vi "reward_behavior_michelle_visjitter_conswinAdapt_enticefx_TSLog_VF_forrecording.vi"() -> ()   [LabVIEW 2019]
doc: "The myRIO Project template acquires acceleration data from the onboard accelerometer and displays the changes of acceleration values in a waveform chart."
uses:
  <vilib>/Analysis/Matrix/Datatypes/RealMatrix.ctl
  <vilib>/myRIO/Instrument Drivers/Onboard IO/DIO/typedefs/DIO Reference.ctl
  <vilib>/myRIO/Common/Instrument Driver Framework/Utilities/typedefs/myRIO Generic Hardware Reference.ctl
  <vilib>/myRIO/Common/Instrument Driver Framework/Utilities/typedefs/Hardware Version Enum.ctl
  <vilib>/myRIO/Common/Instrument Driver Framework/Utilities/typedefs/myRIO v1.0 Reference.ctl
  <vilib>/myRIO/Common/Instrument Driver Framework/Utilities/typedefs/Generic FPGA Reference.ctl
  <vilib>/myRIO/Common/Instrument Driver Framework/myRIO v1.0/DIO/typedefs/DIO Channels List.ctl
  <vilib>/myRIO/Common/Instrument Driver Framework/myRIO v1.0/DIO/typedefs/DIO Channels Enum.ctl
  <vilib>/userdefined/High Color/nirio_resource_hc.ctl
  <vilib>/myRIO/Common/Instrument Driver Framework/myRIO v1.0/Encoder/typedefs/Encoder Signal Mode.ctl
  <vilib>/myRIO/Instrument Drivers/Onboard IO/Encoder/typedefs/Encoder Reference.ctl
  <vilib>/myRIO/Common/Instrument Driver Framework/myRIO v1.0/Encoder/typedefs/Encoder Channels Enum.ctl
  <vilib>/myRIO/Common/Instrument Driver Framework/myRIO v1.0/Encoder/typedefs/Encoder Configuration v1.0.ctl
  <vilib>/myRIO/Common/Instrument Driver Framework/Utilities/vis/Is FPGA Ref Available.vi
  <vilib>/myRIO/Common/Instrument Driver Framework/myRIO v1.0/DIO/vis/myRIO v1.1 Open DIO.vi
  <vilib>/myRIO/Instrument Drivers/Onboard IO/DIO/vis/Write.vi
  <vilib>/myRIO/Common/Instrument Driver Framework/myRIO v1.0/Encoder/vis/myRIO v1.1 Open Encoder.vi
  <vilib>/myRIO/Instrument Drivers/Onboard IO/Encoder/vis/Read.vi
  <vilib>/myRIO/Instrument Drivers/Onboard IO/DIO/vis/Read.vi
  <vilib>/myRIO/Common/Instrument Driver Framework/Utilities/vis/Validate Channels.vi
  <vilib>/myRIO/Common/Instrument Driver Framework/myRIO v1.0/DIO/vis/myRIO v1.0 Reserve DIO.vi
  <vilib>/myRIO/Common/Instrument Driver Framework/myRIO v1.0/Encoder/vis/myRIO v1.0 Reserve Encoder.vi
  <vilib>/myRIO/Common/Instrument Driver Framework/myRIO v1.0/Resource Manager/vis/myRIO v1.0 Reserve Channel List.vi
  <vilib>/myRIO/Common/Instrument Driver Framework/myRIO v1.0/DIO/vis/myRIO v1.0 Build MUX Configuration DIO.vi
  <vilib>/myRIO/Common/Instrument Driver Framework/myRIO v1.0/Encoder/vis/myRIO v1.0 Build MUX Configuration Encoder.vi
  <vilib>/myRIO/Common/Instrument Driver Framework/myRIO v1.0/Resource Manager/vis/myRIO v1.0 Reserve Channel.vi
  <vilib>/myRIO/Common/Instrument Driver Framework/myRIO v1.0/Resource Manager/vis/myRIO v1.0 Unreserve Channel.vi
  <vilib>/myRIO/Common/Instrument Driver Framework/myRIO v1.0/Resource Manager/vis/myRIO v1.0 Create Configuration List.vi
  <vilib>/myRIO/Common/Instrument Driver Framework/myRIO v1.0/Resource Manager/vis/myRIO v1.0 Build Mutex Name.vi
  <vilib>/Utility/VariantDataType/GetNumericInfo.vi
  <vilib>/Utility/error.llb/Error Cluster From Error Code.vi
  <vilib>/myRIO/Common/Instrument Driver Framework/myRIO v1.0/myRIO v1.1 Open.vi
  <vilib>/myRIO/Common/Instrument Driver Framework/Utilities/vis/IO Manager.vi
  <vilib>/myRIO/Common/Instrument Driver Framework/Utilities/vis/Configuration Manager.vi
  <vilib>/myRIO/Common/Instrument Driver Framework/myRIO v1.0/Resource Manager/vis/myRIO v1.0 Configure IO.vi
  <vilib>/myRIO/Common/Instrument Driver Framework/myRIO v1.0/myRIO v1.0 Close.vi
  <vilib>/myRIO/Common/Instrument Driver Framework/myRIO v1.0/Encoder/vis/myRIO v1.0 Configure Encoder.vi
  <vilib>/myRIO/Common/Instrument Driver Framework/myRIO v1.0/Encoder/vis/myRIO v1.0 Read Encoder.vi
  <vilib>/myRIO/Common/Instrument Driver Framework/myRIO v1.0/DIO/vis/myRIO v1.0 Write DIO.vi
  <vilib>/myRIO/Common/Instrument Driver Framework/myRIO v1.0/DIO/vis/myRIO v1.0 Read DIO.vi
  <vilib>/myRIO/Express VI/Onboard IO/Encoder/Encoder Express VI.xnode
  <vilib>/myRIO/Instrument Drivers/Onboard IO/Encoder/vis/myRIO Encoder Open.xnode
  <vilib>/myRIO/Express VI/Onboard IO/DO/DO Express VI.xnode
  <vilib>/myRIO/Instrument Drivers/Onboard IO/DIO/vis/myRIO DIO Open.xnode
  <vilib>/myRIO/Express VI/Onboard IO/DI/DI Express VI.xnode
  <vilib>/myRIO/Instrument Drivers/Onboard IO/Encoder/Encoder.lvlib
  <vilib>/myRIO/Instrument Drivers/Onboard IO/DIO/DIO.lvlib
  <vilib>/Analysis/Matrix/NI_Matrix.lvlib
panel:
  out "AutoEnticeLimit":i32=1000
  out "GetVidFrame":i32
  out "VidTS":dbl[][](array[numeric])
  out "EntTS":dbl[][](array[numeric])
  out "TimeLag":dbl
  out "Lag2":dbl
  out "TestTime":dbl
  out "RewTS":dbl[][](array[numeric])
  out "ConsTS":dbl[][](array[numeric])
  out "LickTS":dbl[][](array[numeric])
  out "ContrastChoice":dbl
  out "Its":i32
  out "BurstCriteria":dbl
  out "LickBurst 2":bool
  out "LickBurst":bool
  out "Enticements":i32
  in  "Entice":bool
  out "Misses":i32
  out "GoAhead":bool
  out "TimeOutDuration":i32
  out "ActiveTime":dbl
  out "ConsumptionGo":bool=TRUE
  out "Consumption_Period":i32
  out "Watch_Display":bool=TRUE
  in  "Give reward":bool
  out "Timings":dbl[](array[numeric])
  out "ISI":dbl
  out "ISI start time":dbl
  out "Time_out":bool=TRUE
  out "Time since lick":dbl
  out "Time of last lick":dbl
  out "Rewarded trials":dbl[](array[numeric])
  out "Rewards":u16
  out "Active Trial":bool
  out "Array temp2":T1
  out "Stimuli Loaded":bool
  out "Stim_ID":dbl[](array[numeric])
  out "Reward_mat":dbl[](array[numeric])
  out "Reward":bool=TRUE
  out "Frame clock":i32
  out "Licks":u32
  out "Lick":bool
  out "Time":dbl
  out "Stop":bool
  in  "Frames to collect":u32
  out "Overflow?":bool
  out "Counter Value":i32
  out "Velocity":dbl
  out "Velocity Plot":dbl[](graph)
  out "Velocity array":dbl[](array[numeric])
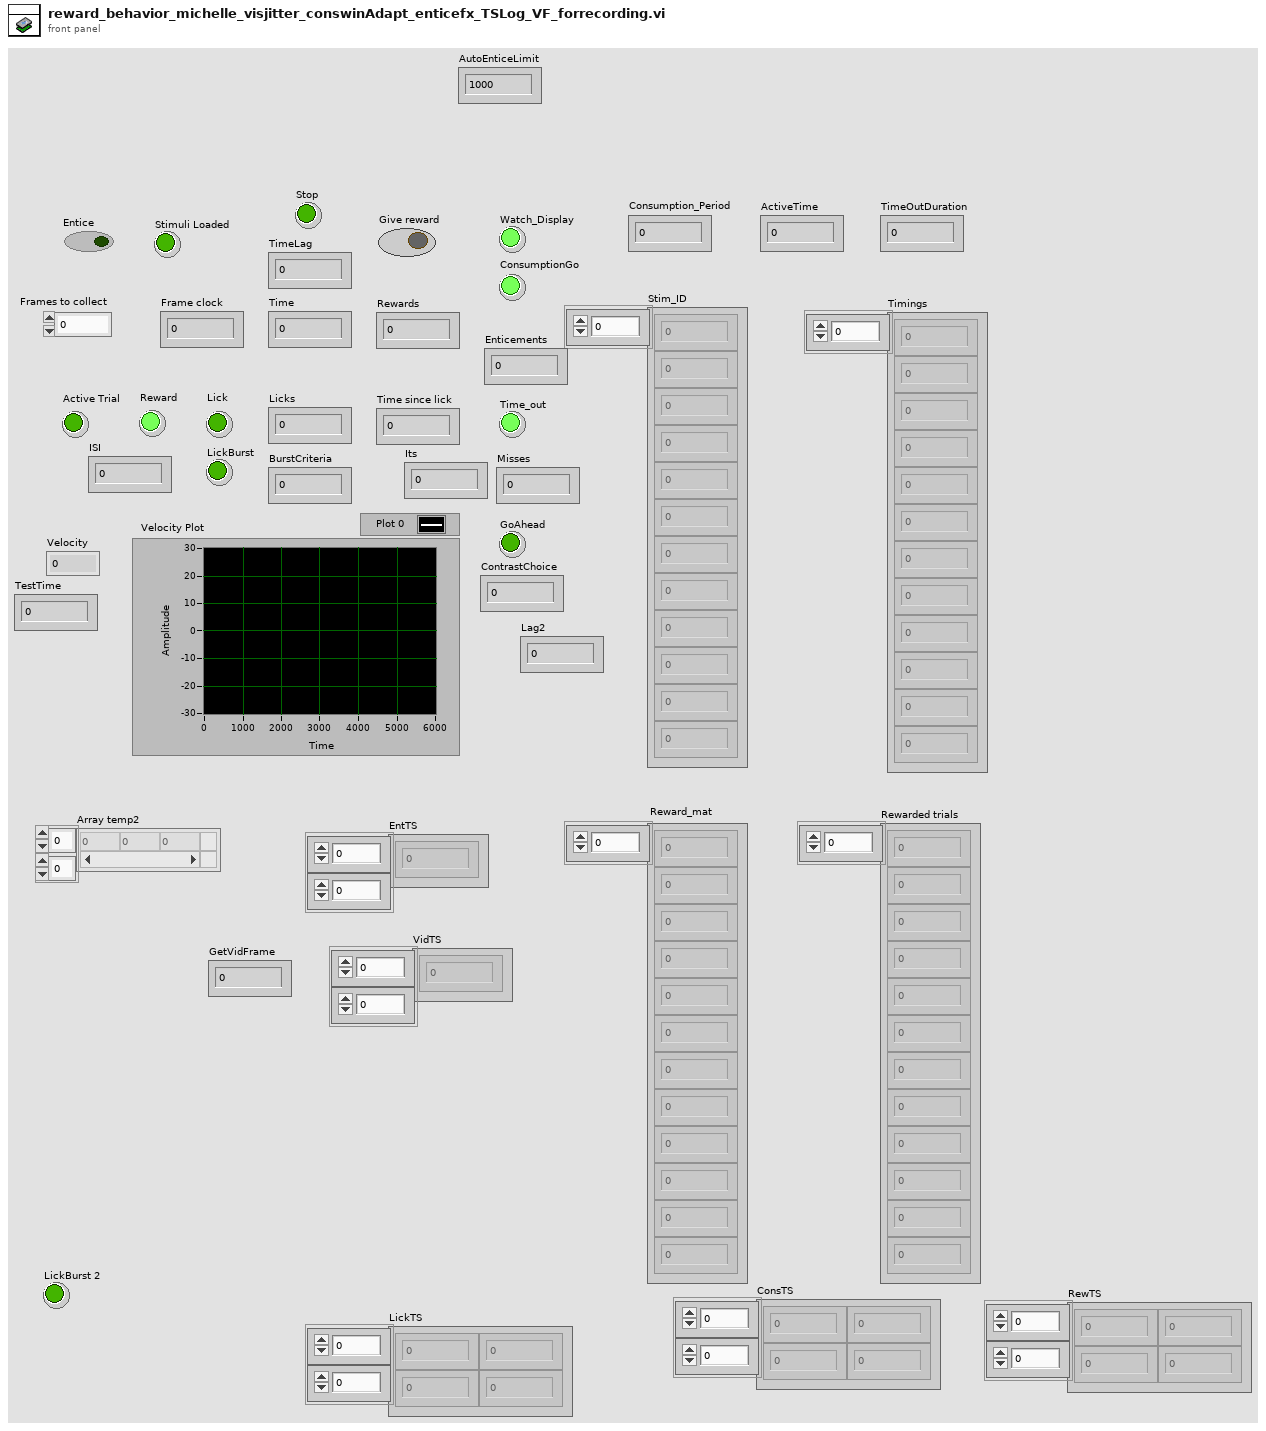
[diagram p1: front panel]
types:
  T1 = typedef "NI_Matrix.lvlib/RealMatrix.ctl" = dbl[][]
  T2 = typedef "DIO.lvlib/DIO Reference.ctl" = cluster{"myRIO Reference":T3, "DIO Channels List":T7}
  T3 = typedef "myRIO Generic Hardware Reference.ctl" = cluster{"myRIO Model":T4, "myRIO Hardware Reference":T5}
  T4 = typedef "Hardware Version Enum.ctl" = enum16{"Unknown", "myRIO-1900", "myRIO-1950", "roboRIO", "NI ELVIS RIO CM", "ELVIS III"}
  T5 = typedef "myRIO v1.0 Reference.ctl" = cluster{"Generic FPGA Reference":T6, "Allow multiple opens":bool}
  T6 = typedef "Generic FPGA Reference.ctl" = refnum<k20>
  T7 = typedef "DIO Channels List.ctl" = T8[]
  T8 = typedef "DIO Channels Enum.ctl" = enum16{"Not Connected", "C/DIO0", "C/DIO1", "C/DIO2", "C/DIO3", "C/DIO4", "C/DIO5", "C/DIO6", "C/DIO7", "A/DIO0", "A/DIO1", "A/DIO2", "A/DIO3", "A/DIO4", "A/DIO5", "A/DIO6", "A/DIO7", "A/DIO8", "A/DIO9", "A/DIO10", "A/DIO11", "A/DIO12", "A/DIO13", "A/DIO14", "A/DIO15", "A/DIO16", "A/DIO17", "A/DIO18", "A/DIO19", "B/DIO0", "B/DIO1", "B/DIO2", "B/DIO3", "B/DIO4", "B/DIO5", "B/DIO6", "B/DIO7", "B/DIO8", "B/DIO9", "B/DIO10", "B/DIO11", "B/DIO12", "B/DIO13", "B/DIO14", "B/DIO15", "B/DIO16", "B/DIO17", "B/DIO18", "B/DIO19", "LED0", "LED1", "LED2", "LED3", "Button0", "DIO/DIO0", "DIO/DIO1", "DIO/DIO2", "DIO/DIO3", "DIO/DIO4", "DIO/DIO5", "DIO/DIO6", "DIO/DIO7", "DIO/DIO8", "DIO/DIO9", "SPI/CS0", "SPI/CS1", "SPI/CS2", "SPI/CS3", "LED RADIO (Green)", "LED RADIO (Red)", "LED COMM (Green)", "LED COMM (Red)", "LED MODE (Green)", "LED MODE (Red)"}
  T9 = typedef "nirio_resource_hc.ctl" = tag
  T10 = typedef "Encoder.lvlib/Encoder Reference.ctl" = cluster{"myRIO Reference":T3, "Encoder Channels Enum":T11}
  T11 = typedef "Encoder Channels Enum.ctl" = enum16{"Not Connected", "C/ENC0", "C/ENC1", "A/ENC", "A/ENC0", "A/ENC1", "A/ENC2", "A/ENC3", "A/ENC4", "A/ENC5", "A/ENC6", "A/ENC7", "A/ENC8", "A/ENC9", "B/ENC", "B/ENC0", "B/ENC1", "B/ENC2", "B/ENC3", "B/ENC4", "B/ENC5", "B/ENC6", "B/ENC7", "B/ENC8", "B/ENC9", "DIO/ENC0", "DIO/ENC1", "DIO/ENC2", "DIO/ENC3", "DIO/ENC4"}
  T12 = typedef "Encoder Signal Mode.ctl" = enum16{"Quadrature phase signal", "Step and direction signal"}
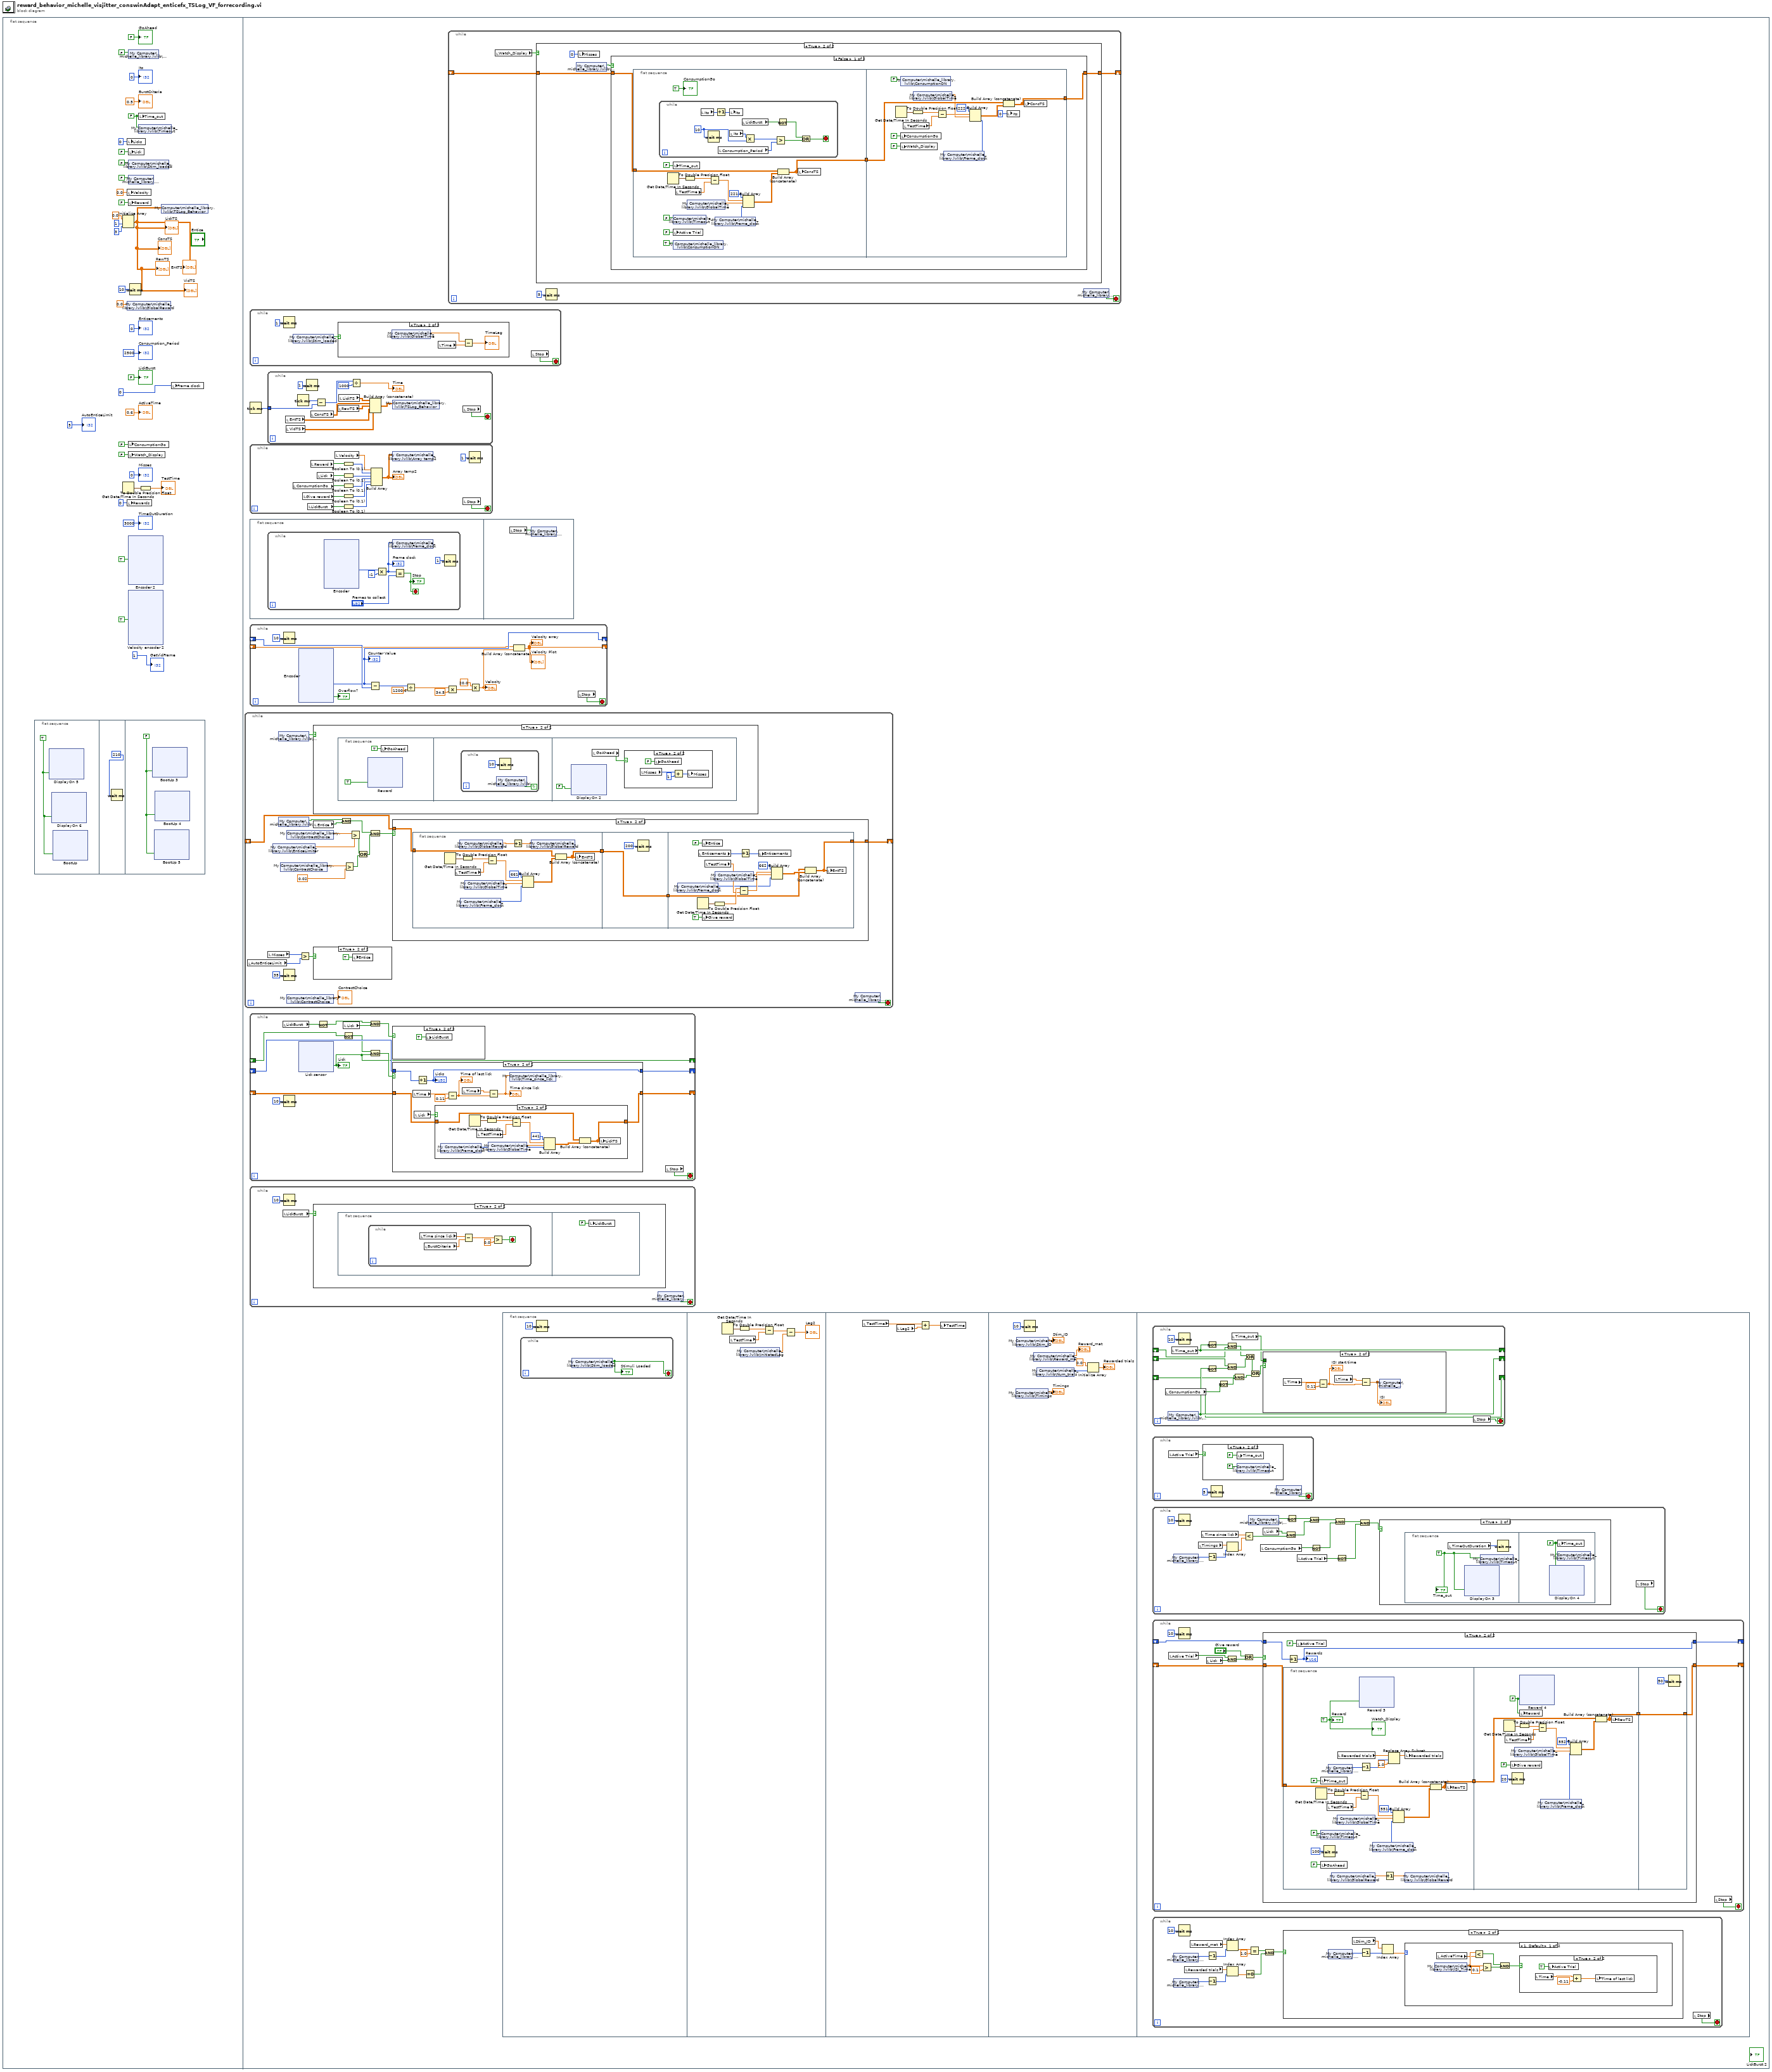
[diagram p0: block diagram]
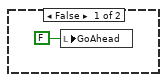
[diagram p6: hidden frame]
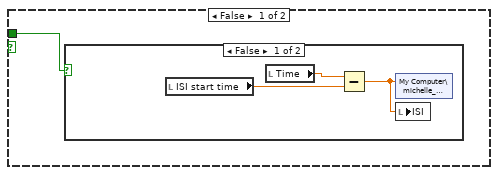
[diagram p12: hidden frame]
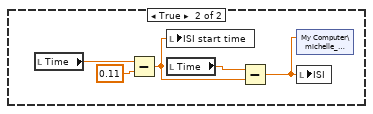
[diagram p13: hidden frame]
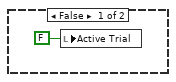
[diagram p14: hidden frame]
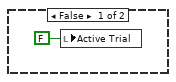
[diagram p15: hidden frame]
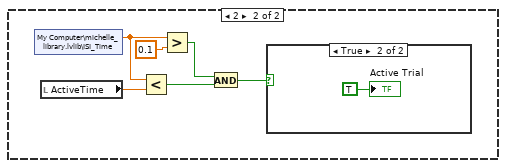
[diagram p16: hidden frame]
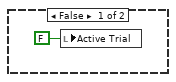
[diagram p17: hidden frame]
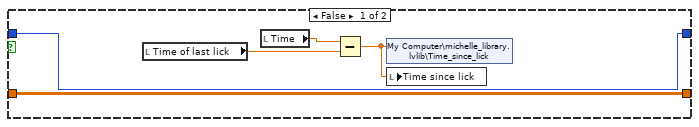
[diagram p20: hidden frame]
diagram:
  n1 = flat-sequence {
    frame #0 {
      w22 = FALSE ("Time_out")
      n2 = flat-sequence {
        frame #0 {
          w34 = TRUE
          n3 = xnode "DisplayOn 5"("C/DIO2 (DIO2)"=w34) -> ()  [unwired: 1 in, 1 out]
          n4 = xnode "DisplayOn 6"("C/DIO1 (DIO1)"=w34) -> ()  [unwired: 1 in, 1 out]
          n5 = xnode "BootUp"("C/DIO3 (DIO3)"=w34) -> ()  [unwired: 1 in, 1 out]
        }
        frame #1 {
          n6 = Wait (ms)(milliseconds to wait=210) -> ()  [unwired: 1 out]
        }
        frame #2 {
          w141 = FALSE
          n7 = xnode "BootUp 3"("C/DIO2 (DIO2)"=w141) -> ()  [unwired: 1 in, 1 out]
          n8 = xnode "BootUp 5"("C/DIO3 (DIO3)"=w141) -> ()  [unwired: 1 in, 1 out]
          n9 = xnode "BootUp 4"("C/DIO1 (DIO1)"=w141) -> ()  [unwired: 1 in, 1 out]
        }
      }
      n10 = Get Date/Time In Seconds() -> (seconds since 1Jan1904=w6:timestamp)
      n11 = Initialize Array(0.0, 1, 3) -> (w3:dbl[][])
      "LickTS" <- w3
      "ConsTS" <- w3
      "RewTS" <- w3
      "EntTS" <- w3
      "VidTS" <- w3
      n12 = local write "Licks"(u32 0 ("Licks")) -> ()
      n13 = local write "Velocity"(0.0 ("Velocity")) -> ()
      n14 = shared-variable "My Computer\\michelle_library.lvlib\\GlobalReward"(0.0) -> ()  [unwired: 1 in, 1 out]
      n15 = local write "Rewards"(u16 0 ("Rewards")) -> ()
      n16 = shared-variable "My Computer\\michelle_library.lvlib\\Display"(FALSE ("Display")) -> ()  [unwired: 1 in, 1 out]
      n17 = local write "Lick"(FALSE ("Lick")) -> ()
      n18 = shared-variable "My Computer\\michelle_library.lvlib\\Stim_loaded"(FALSE ("Stim_loaded")) -> ()  [unwired: 1 in, 1 out]
      n19 = shared-variable "My Computer\\michelle_library.lvlib\\Stop"(FALSE ("Stop")) -> ()  [unwired: 1 in, 1 out]
      n20 = local write "Reward"(FALSE ("Give reward")) -> ()
      n21 = local write "ConsumptionGo"(FALSE ("ConsumptionGo")) -> ()
      n22 = local write "Watch_Display"(FALSE ("Watch_Display")) -> ()
      n23 = xnode "Encoder 2"("Reset Counter"=TRUE) -> ()  [unwired: 1 in, 4 out]
      n24 = xnode "Velocity encoder 2"("Reset Counter"=TRUE) -> ()  [unwired: 1 in, 4 out]
      n25 = Wait (ms)(milliseconds to wait=u32 10) -> ()  [unwired: 1 out]
      n26 = local write "Time_out"(w22) -> ()
      n27 = shared-variable "My Computer\\michelle_library.lvlib\\Timeout"(w22) -> ()  [unwired: 1 in, 1 out]
      n28 = To Double Precision Float(number=w6) -> (double precision float=→"TestTime":dbl)
      n29 = shared-variable "My Computer\\michelle_library.lvlib\\TSLog_Behavior"(w3) -> ()  [unwired: 1 in, 1 out]
      n30 = local write "Frame clock"(u32 0 ("Frames")) -> ()
      "Consumption_Period" <- 2500
      "ActiveTime" <- 0.6
      "TimeOutDuration" <- 3000
      "GoAhead" <- FALSE
      "Misses" <- 0
      "Enticements" <- 0
      "LickBurst" <- FALSE
      "BurstCriteria" <- 0.5
      "Its" <- 0
      "GetVidFrame" <- 1
      "AutoEnticeLimit" <- 5
    }
    frame #1 {
      n31 = while {
        shift-right: [w363] -> _
        shift-left: _ -> [w364]
        stop <- w374 stop-if-true
        n32 = local read "AutoEnticeLimit"() -> (w355:i32)
        n33 = local read "Misses"() -> (w356:i32)
        n34 = shared-variable "My Computer\\michelle_library.lvlib\\EnticeLimiter"() -> (w362:dbl)  [unwired: 1 in, 1 out]
        n35 = shared-variable "My Computer\\michelle_library.lvlib\\Display"() -> (w373:bool)  [unwired: 1 in, 1 out]
        n36 = shared-variable "My Computer\\michelle_library.lvlib\\Display"() -> (w371:bool)  [unwired: 1 in, 1 out]
        n37 = shared-variable "My Computer\\michelle_library.lvlib\\ContrastChoice"() -> (w358:dbl)  [unwired: 1 in, 1 out]
        n38 = Wait (ms)(milliseconds to wait=35) -> ()  [unwired: 1 out]
        n39 = shared-variable "My Computer\\michelle_library.lvlib\\ContrastChoice"() -> (w367:dbl)  [unwired: 1 in, 1 out]
        n40 = shared-variable "My Computer\\michelle_library.lvlib\\ContrastChoice"() -> (→"ContrastChoice":dbl)  [unwired: 1 in, 1 out]
        n41 = Greater?(x=w356, y=w355) -> (0:w372:bool)
        n42 = case shown="True" w373 {
          frame False {
            n43 = local write "GoAhead"(FALSE) -> ()
          }
          frame True {
            n44 = flat-sequence {
              frame #0 {
                n45 = xnode "Reward"("C/DIO2 (DIO2)"=TRUE) -> ()  [unwired: 1 in, 1 out]
                n46 = local write "GoAhead"(TRUE) -> ()
              }
              frame #1 {
                n47 = while {
                  stop <- w448 continue-if-true
                  n48 = shared-variable "My Computer\\michelle_library.lvlib\\Display"() -> (w448:bool)  [unwired: 1 in, 1 out]
                  n49 = Wait (ms)(milliseconds to wait=10) -> ()  [unwired: 1 out]
                }
              }
              frame #2 {
                n50 = xnode "DisplayOn 2"("C/DIO2 (DIO2)"=FALSE) -> ()  [unwired: 1 in, 1 out]
                n51 = local read "GoAhead"() -> (w450:bool)
                n52 = case shown="True" w450 {
                  frame False {
                  }
                  frame True {
                    n53 = local read "Misses"() -> (w489:i32)
                    n54 = local write "GoAhead"(FALSE) -> ()
                    n55 = Add(x=w489, y=1) -> (x+y=w487:i32)
                    n56 = local write "Misses"(w487) -> ()
                  }
                }
              }
            }
          }
        }
        n57 = local read "Entice"() -> (w370:bool)
        n58 = case shown="True" w372 {
          frame False {
          }
          frame True {
            n59 = local write "Entice"(TRUE) -> ()
          }
        }
        n60 = And(x=w371, y=w370) -> (x .and. y?=w368:bool)
        n61 = Greater?(x=w358, y=0.02) -> (0:w359:bool)
        n62 = Greater?(x=w367, y=w362) -> (0:w360:bool)
        n63 = Or(x=w360, y=w359) -> (x .or. y?=w361:bool)
        n64 = And(x=w368, y=w361) -> (x .and. y?=w366:bool)
        n65 = case shown="True" w366 {
          tunnel: w364 -> [w375 w379]
          tunnel: [w375 w376] -> w363
          frame False {
          }
          frame True {
            n66 = flat-sequence {
              tunnel: w379 -> [w382]
              tunnel: [w381] -> w378
              tunnel: w378 -> [w392]
              tunnel: [w392] -> w377
              tunnel: w377 -> [w396]
              tunnel: [w395] -> w376
              frame #0 {
                n67 = Get Date/Time In Seconds() -> (seconds since 1Jan1904=w389:timestamp)
                n68 = local read "TestTime"() -> (w384:dbl)
                n69 = shared-variable "My Computer\\michelle_library.lvlib\\GlobalReward"() -> (w391:dbl)  [unwired: 1 in, 1 out]
                n70 = shared-variable "My Computer\\michelle_library.lvlib\\Frame_clock"() -> (w380:u32)  [unwired: 1 in, 1 out]
                n71 = To Double Precision Float(number=w389) -> (double precision float=w388:dbl)
                n72 = shared-variable "My Computer\\michelle_library.lvlib\\GlobalTime"() -> (w383:dbl)  [unwired: 1 in, 1 out]
                n73 = Subtract(x=w388, y=w384) -> (x-y=w387:dbl)
                n74 = Increment(x=w391) -> (x+1=w390:dbl)
                n75 = Build Array(661, w387, w383, w380) -> (w386:T1)
                n76 = shared-variable "My Computer\\michelle_library.lvlib\\GlobalReward"(w390) -> ()  [unwired: 1 in, 1 out]
                n77 = Build Array (concatenate) ("Build Matrix")(w382, w386) -> (w381:T1)
                n78 = local write "EntTS"(w381) -> ()
              }
              frame #1 {
                n79 = Wait (ms)(milliseconds to wait=200) -> ()  [unwired: 1 out]
              }
              frame #2 {
                n80 = shared-variable "My Computer\\michelle_library.lvlib\\Frame_clock"() -> (w394:u32)  [unwired: 1 in, 1 out]
                n81 = Get Date/Time In Seconds() -> (seconds since 1Jan1904=w403:timestamp)
                n82 = local read "Enticements"() -> (w405:i32)
                n83 = local write "Entice"(FALSE) -> ()
                n84 = local write "Give reward"(TRUE) -> ()
                n85 = local read "TestTime"() -> (w397:dbl)
                n86 = To Double Precision Float(number=w403) -> (double precision float=w402:dbl)
                n87 = shared-variable "My Computer\\michelle_library.lvlib\\GlobalTime"() -> (w398:dbl)  [unwired: 1 in, 1 out]
                n88 = Subtract(x=w402, y=w397) -> (x-y=w401:dbl)
                n89 = Increment(x=w405) -> (x+1=w404:i32)
                n90 = local write "Enticements"(w404) -> ()
                n91 = Build Array(662, w401, w398, w394) -> (w400:T1)
                n92 = Build Array (concatenate) ("Build Matrix")(w396, w400) -> (w395:T1)
                n93 = local write "EntTS"(w395) -> ()
              }
            }
          }
        }
        n94 = shared-variable "My Computer\\michelle_library.lvlib\\Stop"() -> (w374:bool)  [unwired: 1 in, 1 out]
      }
      n95 = while {
        stop <- w341 stop-if-true
        n96 = Wait (ms)(milliseconds to wait=u32 1) -> ()  [unwired: 1 out]
        n97 = shared-variable "My Computer\\michelle_library.lvlib\\Stim_loaded"() -> (w342:bool)  [unwired: 1 in, 1 out]
        n98 = case shown="True" w342 {
          frame False {
          }
          frame True {
            n99 = shared-variable "My Computer\\michelle_library.lvlib\\GlobalTime"() -> (w343:dbl)  [unwired: 1 in, 1 out]
            n100 = local read "Time"() -> (w344:dbl)
            n101 = Subtract(x=w343, y=w344) -> (x-y=→"TimeLag":dbl)
          }
        }
        n102 = local read "Stop"() -> (w341:bool)
      }
      n103 = Tick Count (ms)() -> (millisecond timer value=w339:u32)
      n104 = while {
        stop <- w550 stop-if-true
        n105 = local read "ConsumptionGo"() -> (w548:bool)
        n106 = local read "Give reward"() -> (w547:bool)
        n107 = local read "LickBurst"() -> (w544:bool)
        n108 = local read "Reward"() -> (w555:bool)
        n109 = local read "Lick"() -> (w556:bool)
        n110 = local read "Velocity"() -> (w554:dbl)
        n111 = Boolean To (0,1)(Boolean=w555) -> (0, 1=w553:i16)
        n112 = Boolean To (0,1)(Boolean=w556) -> (0, 1=w552:i16)
        n113 = Boolean To (0,1)(Boolean=w548) -> (0, 1=w546:i16)
        n114 = Boolean To (0,1)(Boolean=w547) -> (0, 1=w545:i16)
        n115 = Boolean To (0,1)(Boolean=w544) -> (0, 1=w543:i16)
        n116 = Build Array(w554, w553, w552, w546, w545, w543) -> (w549:T1)
        "Array temp2" <- w549
        n117 = shared-variable "My Computer\\michelle_library.lvlib\\Array temp2"(w549) -> ()  [unwired: 1 in, 1 out]
        n118 = local read "Stop"() -> (w550:bool)
        n119 = Wait (ms)(milliseconds to wait=u32 1) -> ()  [unwired: 1 out]
      }
      n120 = flat-sequence {
        frame #0 {
          n121 = while {
            stop <- w869 stop-if-true
            n122 = xnode "Encoder"() -> ("Counter Value"=w872:i32)  [unwired: 2 in, 3 out]
            n123 = Multiply(x=w872, y=-1) -> (x*y=w868:i32)
            "Frame clock" <- w868
            n124 = shared-variable "My Computer\\michelle_library.lvlib\\Frame_clock"(w868) -> ()  [unwired: 1 in, 1 out]
            n125 = Equal?(x=w868, y="Frames to collect") -> (x = y?=w869:bool)
            "Stop" <- w869
            n126 = Wait (ms)(milliseconds to wait=u32 1) -> ()  [unwired: 1 out]
          }
        }
        frame #1 {
          n127 = local read "Stop"() -> (w920:bool)
          n128 = shared-variable "My Computer\\michelle_library.lvlib\\Stop"(w920) -> ()  [unwired: 1 in, 1 out]
        }
      }
      n129 = while {
        shift-right: [w1007] -> _
        shift-left: _ -> [w1008]
        shift-right: [w999] -> _
        shift-left: _ -> [w998]
        stop <- w997 stop-if-true
        n130 = Wait (ms)(milliseconds to wait=u32 10) -> ()  [unwired: 1 out]
        n131 = xnode "Encoder"() -> ("Counter Value"=w1007:i32, "Overflow?"=→"Overflow?":bool)  [unwired: 2 in, 2 out]
        "Counter Value" <- w1007
        n132 = Subtract(x=w1007, y=w1008) -> (x-y=w1000:i32)
        n133 = Divide(x=w1000, y=1200.0 ("600")) -> (x/y=w1005:dbl)
        n134 = Multiply(x=w1005, y=34.5) -> (x*y=w1003:dbl)
        n135 = Multiply(x=20.0, y=w1003) -> (x*y=w1001:dbl)
        "Velocity" <- w1001
        n136 = Build Array (concatenate)(w998, w1001) -> (w999:dbl[])
        "Velocity Plot" <- w999
        "Velocity array" <- w999
        n137 = local read "Stop"() -> (w997:bool)
      }
      n138 = while {
        shift-right: [w933] -> _
        shift-left: _ -> [w932]
        shift-right: [w927] -> _
        shift-left: _ -> [w930]
        shift-right: [w921] -> _
        shift-left: _ -> [w922]
        stop <- w931 stop-if-true
        n139 = local read "LickBurst"() -> (w924:bool)
        n140 = Wait (ms)(milliseconds to wait=u32 10) -> ()  [unwired: 1 out]
        n141 = xnode "Lick sensor"() -> ("C/DIO1 (DIO1)"=w927:bool)  [unwired: 1 in, 1 out]
        "Lick" <- w927
        n142 = Not(x=w924) -> (.not. x?=w923:bool)
        n143 = Not(x=w930) -> (.not. x?=w929:bool)
        n144 = local read "Lick"() -> (w925:bool)
        n145 = And(x=w923, y=w925) -> (x .and. y?=w926:bool)
        n146 = And(x=w929, y=w927) -> (x .and. y?=w928:bool)
        n147 = case shown="True" w926 {
          frame False {
          }
          frame True {
            n148 = local write "LickBurst"(TRUE) -> ()
          }
        }
        n149 = case shown="True" w928 {
          tunnel: [w940 w950] -> w933
          tunnel: w932 -> [w940 w949]
          tunnel: w922 -> [w936 w941]
          tunnel: [w936 w943] -> w921
          frame False {
            n150 = local read "Time of last lick"() -> (w938:dbl)
            n151 = local read "Time"() -> (w939:dbl)
            n152 = Subtract(x=w939, y=w938) -> (x-y=w937:dbl)
            n153 = shared-variable "My Computer\\michelle_library.lvlib\\Time_since_lick"(w937) -> ()  [unwired: 1 in, 1 out]
            n154 = local write "Time since lick"(w937) -> ()
          }
          frame True {
            n155 = local read "Time"() -> (w946:dbl)
            n156 = local read "Lick"() -> (w942:bool)
            n157 = Increment(x=w949) -> (x+1=w950:u32)
            "Licks" <- w950
            n158 = case shown="True" w942 {
              tunnel: w941 -> [w951 w957]
              tunnel: [w951 w956] -> w943
              frame False {
              }
              frame True {
                n159 = shared-variable "My Computer\\michelle_library.lvlib\\Frame_clock"() -> (w952:u32)  [unwired: 1 in, 1 out]
                n160 = Get Date/Time In Seconds() -> (seconds since 1Jan1904=w959:timestamp)
                n161 = local read "TestTime"() -> (w954:dbl)
                n162 = To Double Precision Float(number=w959) -> (double precision float=w955:dbl)
                n163 = shared-variable "My Computer\\michelle_library.lvlib\\GlobalTime"() -> (w953:dbl)  [unwired: 1 in, 1 out]
                n164 = Subtract(x=w955, y=w954) -> (x-y=w960:dbl)
                n165 = Build Array(441, w960, w953, w952) -> (w961:T1)
                n166 = Build Array (concatenate) ("Build Matrix")(w957, w961) -> (w956:T1)
                n167 = local write "LickTS"(w956) -> ()
              }
            }
            n168 = Subtract(x=w946, y=0.11) -> (x-y=w944:dbl)
            "Time of last lick" <- w944
            n169 = local read "Time"() -> (w948:dbl)
            n170 = Subtract(x=w948, y=w944) -> (x-y=w947:dbl)
            "Time since lick" <- w947
            n171 = shared-variable "My Computer\\michelle_library.lvlib\\Time_since_lick"(w947) -> ()  [unwired: 1 in, 1 out]
          }
        }
        n172 = local read "Stop"() -> (w931:bool)
      }
      n173 = while {
        stop <- w348 stop-if-true
        n174 = local read "LickBurst"() -> (w346:bool)
        n175 = Wait (ms)(milliseconds to wait=u32 10) -> ()  [unwired: 1 out]
        n176 = case shown="True" w346 {
          frame False {
          }
          frame True {
            n177 = flat-sequence {
              frame #0 {
                n178 = while {
                  stop <- w351 stop-if-true
                  n179 = local read "Time since lick"() -> (w352:dbl)
                  n180 = local read "BurstCriteria"() -> (w353:dbl)
                  n181 = Subtract(x=w352, y=w353) -> (x-y=w349:dbl)
                  n182 = Greater?(x=w349, y=0.0) -> (0:w351:bool)
                }
              }
              frame #1 {
                n183 = local write "LickBurst"(FALSE) -> ()
              }
            }
          }
        }
        n184 = shared-variable "My Computer\\michelle_library.lvlib\\Stop"() -> (w348:bool)  [unwired: 1 in, 1 out]
      }
      n185 = while {
        tunnel: w339 -> [w1068]
        stop <- w1066 stop-if-true
        n186 = local read "EntTS"() -> (w1058:dbl[][])
        n187 = local read "VidTS"() -> (w1057:dbl[][])
        n188 = Tick Count (ms)() -> (millisecond timer value=w1069:u32)
        n189 = Wait (ms)(milliseconds to wait=u32 1) -> ()  [unwired: 1 out]
        n190 = local read "ConsTS"() -> (w1061:dbl[][])
        n191 = Subtract(x=w1069, y=w1068) -> (x-y=w1065:u32)
        n192 = local read "RewTS"() -> (w1060:dbl[][])
        n193 = local read "LickTS"() -> (w1062:dbl[][])
        n194 = Divide(x=w1065, y=u32 1000) -> (x/y=→"Time":dbl)
        n195 = Build Array (concatenate) ("Build Matrix")(w1062, w1061, w1060, w1058, w1057) -> (w1059:T1)
        n196 = shared-variable "My Computer\\michelle_library.lvlib\\TSLog_Behavior"(w1059) -> ()  [unwired: 1 in, 1 out]
        n197 = local read "Stop"() -> (w1066:bool)
      }
      n198 = while {
        shift-right: [w490] -> _
        shift-left: _ -> [w491]
        stop <- w494 stop-if-true
        n199 = local read "Watch_Display"() -> (w493:bool)
        n200 = case shown="True" w493 {
          tunnel: w491 -> [w495 w497]
          tunnel: [w495 w496] -> w490
          frame False {
          }
          frame True {
            n201 = shared-variable "My Computer\\michelle_library.lvlib\\Display"() -> (w499:bool)  [unwired: 1 in, 1 out]
            n202 = local write "Misses"(0) -> ()
            n203 = case shown="False" w499 {
              tunnel: w497 -> [w502 w542]
              tunnel: [w500 w542] -> w496
              frame False {
                n204 = flat-sequence {
                  tunnel: w502 -> [w506]
                  tunnel: [w505] -> w501
                  tunnel: w501 -> [w532]
                  tunnel: [w531] -> w500
                  frame #0 {
                    n205 = while {
                      stop <- w521 stop-if-true
                      w522 = 10
                      n206 = local read "Its"() -> (w526:i32)
                      n207 = Wait (ms)(milliseconds to wait=w522) -> ()  [unwired: 1 out]
                      n208 = Increment(x=w526) -> (x+1=w525:i32)
                      n209 = local read "Consumption_Period"() -> (w519:i32)
                      n210 = local write "Its"(w525) -> ()
                      n211 = local read "Its"() -> (w523:i32)
                      n212 = local read "LickBurst"() -> (w527:bool)
                      n213 = Multiply(x=w523, y=w522) -> (x*y=w520:i32)
                      n214 = Greater?(x=w520, y=w519) -> (0:w518:bool)
                      n215 = Not(x=w527) -> (.not. x?=w524:bool)
                      n216 = Or(x=w524, y=w518) -> (x .or. y?=w521:bool)
                    }
                    n217 = Get Date/Time In Seconds() -> (seconds since 1Jan1904=w511:timestamp)
                    n218 = local write "Time_out"(FALSE) -> ()
                    n219 = shared-variable "My Computer\\michelle_library.lvlib\\Timeout"(FALSE) -> ()  [unwired: 1 in, 1 out]
                    n220 = local write "Active Trial"(FALSE) -> ()
                    n221 = shared-variable "My Computer\\michelle_library.lvlib\\ConsumptionON"(TRUE) -> ()  [unwired: 1 in, 1 out]
                    n222 = local read "TestTime"() -> (w508:dbl)
                    n223 = To Double Precision Float(number=w511) -> (double precision float=w509:dbl)
                    n224 = shared-variable "My Computer\\michelle_library.lvlib\\GlobalTime"() -> (w504:dbl)  [unwired: 1 in, 1 out]
                    n225 = Subtract(x=w509, y=w508) -> (x-y=w512:dbl)
                    n226 = shared-variable "My Computer\\michelle_library.lvlib\\Frame_clock"() -> (w503:u32)  [unwired: 1 in, 1 out]
                    n227 = Build Array(221, w512, w504, w503) -> (w507:T1)
                    n228 = Build Array (concatenate) ("Build Matrix")(w506, w507) -> (w505:T1)
                    n229 = local write "ConsTS"(w505) -> ()
                    "ConsumptionGo" <- TRUE
                  }
                  frame #1 {
                    n230 = Get Date/Time In Seconds() -> (seconds since 1Jan1904=w536:timestamp)
                    n231 = shared-variable "My Computer\\michelle_library.lvlib\\ConsumptionON"(FALSE) -> ()  [unwired: 1 in, 1 out]
                    n232 = local write "ConsumptionGo"(FALSE ("ConsumptionGo")) -> ()
                    n233 = local write "Watch_Display"(FALSE ("Watch_Display")) -> ()
                    n234 = local read "TestTime"() -> (w533:dbl)
                    n235 = To Double Precision Float(number=w536) -> (double precision float=w534:dbl)
                    n236 = shared-variable "My Computer\\michelle_library.lvlib\\GlobalTime"() -> (w529:dbl)  [unwired: 1 in, 1 out]
                    n237 = Subtract(x=w534, y=w533) -> (x-y=w537:dbl)
                    n238 = shared-variable "My Computer\\michelle_library.lvlib\\Frame_clock"() -> (w528:u32)  [unwired: 1 in, 1 out]
                    n239 = Build Array(222, w537, w529, w528) -> (w530:T1)
                    n240 = Build Array (concatenate) ("Build Matrix")(w532, w530) -> (w531:T1)
                    n241 = local write "Its"(0) -> ()
                    n242 = local write "ConsTS"(w531) -> ()
                  }
                }
              }
              frame True {
              }
            }
          }
        }
        n243 = Wait (ms)(milliseconds to wait=u32 5) -> ()  [unwired: 1 out]
        n244 = shared-variable "My Computer\\michelle_library.lvlib\\Stop"() -> (w494:bool)  [unwired: 1 in, 1 out]
      }
      n245 = flat-sequence {
        frame #0 {
          n246 = while {
            stop <- w558 stop-if-true
            n247 = shared-variable "My Computer\\michelle_library.lvlib\\Stim_loaded"() -> (w558:bool)  [unwired: 1 in, 1 out]
            "Stimuli Loaded" <- w558
          }
          n248 = Wait (ms)(milliseconds to wait=u32 10) -> ()  [unwired: 1 out]
        }
        frame #1 {
          n249 = Get Date/Time In Seconds() -> (seconds since 1Jan1904=w564:timestamp)
          n250 = local read "TestTime"() -> (w563:dbl)
          n251 = To Double Precision Float(number=w564) -> (double precision float=w562:dbl)
          n252 = shared-variable "My Computer\\michelle_library.lvlib\\InitiatedLag"() -> (w561:dbl)  [unwired: 1 in, 1 out]
          n253 = Subtract(x=w562, y=w563) -> (x-y=w559:dbl)
          n254 = Subtract(x=w559, y=w561) -> (x-y=→"Lag2":dbl)
        }
        frame #2 {
          n255 = local read "TestTime"() -> (w565:dbl)
          n256 = local read "Lag2"() -> (w566:dbl)
          n257 = Add(x=w565, y=w566) -> (x+y=w567:dbl)
          n258 = local write "TestTime"(w567) -> ()
        }
        frame #3 {
          n259 = shared-variable "My Computer\\michelle_library.lvlib\\Timings"() -> (→"Timings":dbl[])  [unwired: 1 in, 1 out]
          n260 = shared-variable "My Computer\\michelle_library.lvlib\\Stim_ID"() -> (→"Stim_ID":dbl[])  [unwired: 1 in, 1 out]
          n261 = Wait (ms)(milliseconds to wait=u32 10) -> ()  [unwired: 1 out]
          n262 = shared-variable "My Computer\\michelle_library.lvlib\\Reward_mat"() -> (→"Reward_mat":dbl[])  [unwired: 1 in, 1 out]
          n263 = shared-variable "My Computer\\michelle_library.lvlib\\Num_trials"() -> (w571:u32)  [unwired: 1 in, 1 out]
          n264 = Initialize Array(0.0 ("element"), w571) -> (→"Rewarded trials":dbl[])
        }
        frame #4 {
          n265 = while {
            shift-right: [w687] -> _
            shift-left: _ -> [w685]
            shift-right: [w683] -> _
            shift-left: _ -> [w682]
            shift-right: [w677] -> _
            shift-left: _ -> [w675]
            stop <- w688 stop-if-true
            n266 = local read "ConsumptionGo"() -> (w677:bool)
            n267 = shared-variable "My Computer\\michelle_library.lvlib\\Display"() -> (w683:bool)  [unwired: 1 in, 1 out]
            n268 = local read "Time_out"() -> (w687:bool)
            n269 = Wait (ms)(milliseconds to wait=u32 10) -> ()  [unwired: 1 out]
            n270 = Not(x=w687) -> (.not. x?=w686:bool)
            n271 = Not(x=w683) -> (.not. x?=w681:bool)
            n272 = Not(x=w677) -> (.not. x?=w678:bool)
            n273 = And(x=w686, y=w685) -> (x .and. y?=w680:bool)
            n274 = And(x=w682, y=w681) -> (x .and. y?=w676:bool)
            n275 = local read "Time_out"() -> (w684:bool)
            n276 = And(x=w675, y=w678) -> (x .and. y?=w674:bool)
            n277 = Or(x=w680, y=w676) -> (x .or. y?=w673:bool)
            n278 = Or(x=w673, y=w674) -> (x .or. y?=w672:bool)
            n279 = case shown="True" w672 {
              tunnel: w684 -> [w689 _]
              frame False {
                n280 = case shown="False" w689 {
                  frame False {
                    n281 = local read "ISI start time"() -> (w692:dbl)
                    n282 = local read "Time"() -> (w691:dbl)
                    n283 = Subtract(x=w691, y=w692) -> (x-y=w690:dbl)
                    n284 = shared-variable "My Computer\\michelle_library.lvlib\\ISI"(w690) -> ()  [unwired: 1 in, 1 out]
                    n285 = local write "ISI"(w690) -> ()
                  }
                  frame True {
                    n286 = local read "Time"() -> (w697:dbl)
                    n287 = Subtract(x=w697, y=0.11) -> (x-y=w694:dbl)
                    n288 = local write "ISI start time"(w694) -> ()
                    n289 = local read "Time"() -> (w695:dbl)
                    n290 = Subtract(x=w695, y=w694) -> (x-y=w693:dbl)
                    n291 = shared-variable "My Computer\\michelle_library.lvlib\\ISI"(w693) -> ()  [unwired: 1 in, 1 out]
                    n292 = local write "ISI"(w693) -> ()
                  }
                }
              }
              frame True {
                n293 = local read "Time"() -> (w702:dbl)
                n294 = Subtract(x=w702, y=0.11) -> (x-y=w699:dbl)
                "ISI start time" <- w699
                n295 = local read "Time"() -> (w700:dbl)
                n296 = Subtract(x=w700, y=w699) -> (x-y=w698:dbl)
                "ISI" <- w698
                n297 = shared-variable "My Computer\\michelle_library.lvlib\\ISI"(w698) -> ()  [unwired: 1 in, 1 out]
              }
            }
            n298 = local read "Stop"() -> (w688:bool)
          }
          n299 = while {
            stop <- w577 stop-if-true
            n300 = local read "Active Trial"() -> (w576:bool)
            n301 = case shown="True" w576 {
              frame False {
              }
              frame True {
                n302 = local write "Time_out"(FALSE) -> ()
                n303 = shared-variable "My Computer\\michelle_library.lvlib\\Timeout"(FALSE) -> ()  [unwired: 1 in, 1 out]
              }
            }
            n304 = Wait (ms)(milliseconds to wait=5) -> ()  [unwired: 1 out]
            n305 = shared-variable "My Computer\\michelle_library.lvlib\\Stop"() -> (w577:bool)  [unwired: 1 in, 1 out]
          }
          n306 = while {
            stop <- w598 stop-if-true
            n307 = shared-variable "My Computer\\michelle_library.lvlib\\Trial"() -> (w588:u32)  [unwired: 1 in, 1 out]
            n308 = Wait (ms)(milliseconds to wait=u32 10) -> ()  [unwired: 1 out]
            n309 = local read "Timings"() -> (w590:dbl[])
            n310 = local read "Time since lick"() -> (w597:dbl)
            n311 = Decrement(x=w588) -> (x-1=w587:u32)
            n312 = Index Array(array=w590, index=w587) -> (element=w589:dbl)
            n313 = Less?(x=w597, y=w589) -> (x < y?=w596:bool)
            n314 = shared-variable "My Computer\\michelle_library.lvlib\\Display"() -> (w593:bool)  [unwired: 1 in, 1 out]
            n315 = local read "ConsumptionGo"() -> (w585:bool)
            n316 = local read "Lick"() -> (w595:bool)
            n317 = And(x=w595, y=w596) -> (x .and. y?=w591:bool)
            n318 = Not(x=w593) -> (.not. x?=w592:bool)
            n319 = local read "Active Trial"() -> (w580:bool)
            n320 = And(x=w592, y=w591) -> (x .and. y?=w584:bool)
            n321 = Not(x=w585) -> (.not. x?=w586:bool)
            n322 = And(x=w584, y=w586) -> (x .and. y?=w582:bool)
            n323 = Not(x=w580) -> (.not. x?=w583:bool)
            n324 = And(x=w582, y=w583) -> (x .and. y?=w581:bool)
            n325 = case shown="True" w581 {
              frame False {
              }
              frame True {
                n326 = flat-sequence {
                  frame #0 {
                    w599 = TRUE
                    n327 = local read "TimeOutDuration"() -> (w600:i32)
                    n328 = xnode "DisplayOn 3"("C/DIO3 (DIO3)"=w599) -> ()  [unwired: 1 in, 1 out]
                    n329 = shared-variable "My Computer\\michelle_library.lvlib\\Timeout"(w599) -> ()  [unwired: 1 in, 1 out]
                    n330 = Wait (ms)(milliseconds to wait=w600) -> ()  [unwired: 1 out]
                    "Time_out" <- w599
                  }
                  frame #1 {
                    w636 = FALSE ("Timeout")
                    n331 = xnode "DisplayOn 4"("C/DIO3 (DIO3)"=w636) -> ()  [unwired: 1 in, 1 out]
                    n332 = local write "Time_out"(w636) -> ()
                    n333 = shared-variable "My Computer\\michelle_library.lvlib\\Timeout"(w636) -> ()  [unwired: 1 in, 1 out]
                  }
                }
              }
            }
            n334 = local read "Stop"() -> (w598:bool)
          }
          n335 = while {
            shift-right: [w749] -> _
            shift-left: _ -> [w748]
            shift-right: [w741] -> _
            shift-left: _ -> [w742]
            stop <- w751 stop-if-true
            n336 = local read "Active Trial"() -> (w746:bool)
            n337 = Wait (ms)(milliseconds to wait=u32 10) -> ()  [unwired: 1 out]
            n338 = local read "Lick"() -> (w747:bool)
            n339 = And(x=w746, y=w747) -> (x .and. y?=w745:bool)
            n340 = Or(x="Give reward", y=w745) -> (x .or. y?=w744:bool)
            n341 = case shown="True" w744 {
              tunnel: [w753 w760] -> w749
              tunnel: w748 -> [w753 w759]
              tunnel: w742 -> [w752 w757]
              tunnel: [w752 w756] -> w741
              frame False {
              }
              frame True {
                n342 = flat-sequence {
                  tunnel: w757 -> [w766]
                  tunnel: [w763] -> w754
                  tunnel: [w822] -> w755
                  tunnel: w754 -> [w820]
                  tunnel: [w866] -> w756
                  tunnel: w755 -> [w866]
                  frame #0 {
                    w781 = TRUE ("C/DIO0 (DIO0)")
                    n343 = Get Date/Time In Seconds() -> (seconds since 1Jan1904=w770:timestamp)
                    n344 = local write "Time_out"(FALSE) -> ()
                    n345 = shared-variable "My Computer\\michelle_library.lvlib\\Timeout"(FALSE) -> ()  [unwired: 1 in, 1 out]
                    n346 = local write "GoAhead"(FALSE) -> ()
                    n347 = Wait (ms)(milliseconds to wait=u32 100) -> ()  [unwired: 1 out]
                    n348 = local read "TestTime"() -> (w764:dbl)
                    n349 = shared-variable "My Computer\\michelle_library.lvlib\\Trial"() -> (w780:u32)  [unwired: 1 in, 1 out]
                    n350 = shared-variable "My Computer\\michelle_library.lvlib\\GlobalReward"() -> (w772:dbl)  [unwired: 1 in, 1 out]
                    n351 = To Double Precision Float(number=w770) -> (double precision float=w769:dbl)
                    n352 = shared-variable "My Computer\\michelle_library.lvlib\\GlobalTime"() -> (w762:dbl)  [unwired: 1 in, 1 out]
                    n353 = local read "Rewarded trials"() -> (w778:dbl[])
                    n354 = Subtract(x=w769, y=w764) -> (x-y=w768:dbl)
                    n355 = xnode "Reward 3"("C/DIO0 (DIO0)"=w781) -> ()  [unwired: 1 in, 1 out]
                    n356 = Decrement(x=w780) -> (x-1=w779:u32)
                    n357 = shared-variable "My Computer\\michelle_library.lvlib\\Frame_clock"() -> (w761:u32)  [unwired: 1 in, 1 out]
                    n358 = Increment(x=w772) -> (x+1=w771:dbl)
                    n359 = Replace Array Subset(array=w778, new element=1.0 ("new element/subarray"), index=w779) -> (w776:dbl[])
                    n360 = Build Array(551, w768, w762, w761) -> (w767:T1)
                    n361 = local write "Rewarded trials"(w776) -> ()
                    n362 = shared-variable "My Computer\\michelle_library.lvlib\\GlobalReward"(w771) -> ()  [unwired: 1 in, 1 out]
                    n363 = Build Array (concatenate) ("Build Matrix")(w766, w767) -> (w763:T1)
                    n364 = local write "RewTS"(w763) -> ()
                    "Reward" <- w781
                    "Watch_Display" <- w781
                  }
                  frame #1 {
                    w830 = FALSE ("C/DIO0 (DIO0)")
                    n365 = Get Date/Time In Seconds() -> (seconds since 1Jan1904=w827:timestamp)
                    n366 = local read "TestTime"() -> (w821:dbl)
                    n367 = local write "Give reward"(FALSE ("Give reward")) -> ()
                    n368 = Wait (ms)(milliseconds to wait=u32 20) -> ()  [unwired: 1 out]
                    n369 = shared-variable "My Computer\\michelle_library.lvlib\\GlobalTime"() -> (w819:dbl)  [unwired: 1 in, 1 out]
                    n370 = To Double Precision Float(number=w827) -> (double precision float=w826:dbl)
                    n371 = xnode "Reward 4"("C/DIO0 (DIO0)"=w830) -> ()  [unwired: 1 in, 1 out]
                    n372 = local write "Reward"(w830) -> ()
                    n373 = Subtract(x=w826, y=w821) -> (x-y=w825:dbl)
                    n374 = shared-variable "My Computer\\michelle_library.lvlib\\Frame_clock"() -> (w818:u32)  [unwired: 1 in, 1 out]
                    n375 = Build Array(552, w825, w819, w818) -> (w823:T1)
                    n376 = Build Array (concatenate) ("Build Matrix")(w820, w823) -> (w822:T1)
                    n377 = local write "RewTS"(w822) -> ()
                  }
                  frame #2 {
                    n378 = Wait (ms)(milliseconds to wait=u32 50) -> ()  [unwired: 1 out]
                  }
                }
                n379 = Increment(x=w759) -> (x+1=w760:u16)
                "Rewards" <- w760
                n380 = local write "Active Trial"(FALSE ("Active Trial")) -> ()
              }
            }
            n381 = local read "Stop"() -> (w751:bool)
          }
          n382 = while {
            stop <- w716 stop-if-true
            n383 = shared-variable "My Computer\\michelle_library.lvlib\\Trial"() -> (w712:u32)  [unwired: 1 in, 1 out]
            n384 = shared-variable "My Computer\\michelle_library.lvlib\\Trial"() -> (w708:u32)  [unwired: 1 in, 1 out]
            n385 = Wait (ms)(milliseconds to wait=u32 10) -> ()  [unwired: 1 out]
            n386 = local read "Rewarded trials"() -> (w709:dbl[])
            n387 = local read "Reward_mat"() -> (w711:dbl[])
            n388 = Decrement(x=w712) -> (x-1=w713:u32)
            n389 = Decrement(x=w708) -> (x-1=w707:u32)
            n390 = Index Array(array=w711, index=w713) -> (element=w714:dbl)
            n391 = Index Array(array=w709, index=w707) -> (element=w706:dbl)
            n392 = Equal To 0?(x=w706) -> (x = 0?=w705:bool)
            n393 = Equal?(x=w714, y=1.0) -> (x = y?=w704:bool)
            n394 = And(x=w704, y=w705) -> (x .and. y?=w703:bool)
            n395 = case shown="True" w703 {
              frame False {
                n396 = local write "Active Trial"(FALSE ("Active_trial")) -> ()
              }
              frame True {
                n397 = shared-variable "My Computer\\michelle_library.lvlib\\Trial"() -> (w719:u32)  [unwired: 1 in, 1 out]
                n398 = local read "Stim_ID"() -> (w721:dbl[])
                n399 = Decrement(x=w719) -> (x-1=w720:u32)
                n400 = Index Array(array=w721, index=w720) -> (element=w718:dbl)
                n401 = case shown="1, Default" w718 {
                  frame 1, Default {
                    n402 = shared-variable "My Computer\\michelle_library.lvlib\\ISI_Time"() -> (w727:dbl)  [unwired: 1 in, 1 out]
                    n403 = local read "ActiveTime"() -> (w722:dbl)
                    n404 = Less?(x=w727, y=w722) -> (x < y?=w725:bool)
                    n405 = Greater?(x=w727, y=0.1) -> (0:w724:bool)
                    n406 = And(x=w725, y=w724) -> (x .and. y?=w723:bool)
                    n407 = case shown="True" w723 {
                      frame False {
                        n408 = local write "Active Trial"(FALSE ("Active Trial")) -> ()
                      }
                      frame True {
                        n409 = local read "Time"() -> (w731:dbl)
                        n410 = local write "Active Trial"(TRUE ("Active Trial")) -> ()
                        n411 = Add(x=w731, y=-0.11) -> (x+y=w729:dbl)
                        n412 = local write "Time of last lick"(w729) -> ()
                      }
                    }
                  }
                  frame 2 {
                    n413 = shared-variable "My Computer\\michelle_library.lvlib\\ISI_Time"() -> (w737:dbl)  [unwired: 1 in, 1 out]
                    n414 = local read "ActiveTime"() -> (w733:dbl)
                    n415 = Less?(x=w737, y=w733) -> (x < y?=w735:bool)
                    n416 = Greater?(x=w737, y=0.1) -> (0:w736:bool)
                    n417 = And(x=w736, y=w735) -> (x .and. y?=w734:bool)
                    n418 = case shown="True" w734 {
                      frame False {
                        n419 = local write "Active Trial"(FALSE ("Active Trial")) -> ()
                      }
                      frame True {
                        "Active Trial" <- TRUE ("Active Trial")
                      }
                    }
                  }
                }
              }
            }
            n420 = local read "Stop"() -> (w716:bool)
          }
        }
      }
    }
  }
